vi "BfrPkt - Set Buffer Direction.vi"(8 "error in (no error)":errorcluster, 10 "External?":bool, 11 "Node Ptr":T1 format="%.0x") -> (0 "error out":errorcluster, 3 "Node Ptr out":T1 format="%.0x")   [LabVIEW 2019, in "UDP-Custom-Device System Explorer.lvlib"]
uses:
  UDP-Custom-Device System Explorer.lvlib
  <vilib>/NI VeriStand/Custom Device API/Custom Device Item Ref.ctl
  <vilib>/NI VeriStand/Custom Device API/Custom Device Channel Type.ctl
  <vilib>/NI VeriStand/Custom Device API/Custom Device API.lvlib
  <vilib>/NI VeriStand/Custom Device Tools/Custom Device Utility Library/Custom Device Utility Library.lvlib
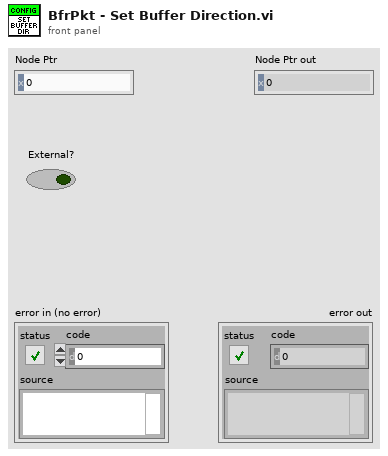
[diagram p1: front panel]
types:
  T1 = typedef "Custom Device API.lvlib/Custom Device Item Ref.ctl" = u64
  T2 = typedef "Custom Device API.lvlib/Custom Device Channel Type.ctl" = enum16{"Input", "Output"}
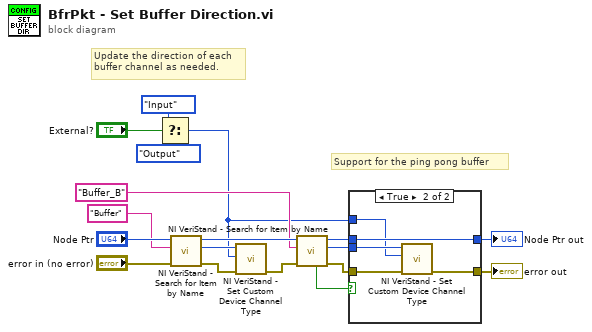
[diagram p0: block diagram]
diagram:
  # "Update the direction of each\nbuffer channel as needed."
  # "Support for the ping pong buffer"
  n1 = Select(t=Custom_Device_Channel_Type."Input" ("Type"), s="External?", f=Custom_Device_Channel_Type."Output" ("Type")) -> (s? t:f=w4:T2)
  n2 = call <vilib>:"NI VeriStand - Search for Item by Name.vi"("error in"="error in (no error)", "Item Name"="Buffer", "Section Ref in"="Node Ptr") -> ("error out"=w17:errorcluster, "Item Ref"=w14:T1, "Section Ref out"=w10:T1)  [unwired: 5 in, 1 out]
  n3 = call <vilib>:"NI VeriStand - Set Custom Device Channel Type.vi"("error in (no error)"=w17, "Type"=w4, "Channel Ref in"=w14) -> ("error out"=w9:errorcluster)  [unwired: 7 in, 1 out]
  n4 = call <vilib>:"NI VeriStand - Search for Item by Name.vi"("error in"=w9, "Item Name"="Buffer_B", "Section Ref in"=w10) -> ("error out"=w2:errorcluster, "Item Ref"=w3:T1, "Section Ref out"=w6:T1, "Found"=w7:bool)  [unwired: 5 in]
  n5 = case shown="True" w7 {
    tunnel: w6 -> [w20 w25]
    tunnel: [w20 w25] -> w5
    tunnel: w4 -> [_ w23]
    tunnel: w3 -> [_ w24]
    tunnel: w2 -> [w19 w22]
    tunnel: [w19 w21] -> w1
    frame False {
    }
    frame True {
      n6 = call <vilib>:"NI VeriStand - Set Custom Device Channel Type.vi"("error in (no error)"=w22, "Type"=w23, "Channel Ref in"=w24) -> ("error out"=w21:errorcluster)  [unwired: 7 in, 1 out]
    }
  }
  "error out" <- w1
  "Node Ptr out" <- w5
